vi "Get Spectrum.vi"(0 "waveform (V)":waveform(dbl), 1 "FFT window (7 Term B-Harris)":T1=8 items=["Rectangle"=0, "Hanning"=1, "Hamming"=2, "Blackman-Harris"=3, "Exact Blackman"=4, "Blackman"=5, "Flat Top"=6, "4 Term B-Harris "=7, "7 Term B-Harris"=8, "Low Sidelobe"=9, "Blackman Nuttall"=11, "Triangle"=30, "Bartlett-Hanning"=31, "Bohman"=32, "Parzen"=33, "Welch"=34, "Kaiser"=60, "Dolph-Chebyshev"=61, "Gaussian"=62], 11 "error in (no error)":errorcluster) -> (4 "power spectrum (dBm)":cluster{"f0":dbl, "df":dbl, "magnitude":dbl[]}, 15 "error out":errorcluster)   [LabVIEW 2021]
uses:
  <vilib>/Analysis/4window.llb/windowTd.ctl
  <vilib>/measure/maspectr.llb/FFT Power Spectrum and PSD for 1 Chan.vi
  <vilib>/measure/NI_MAPro.lvlib
  <vilib>/Analysis/NI_AALPro.lvlib
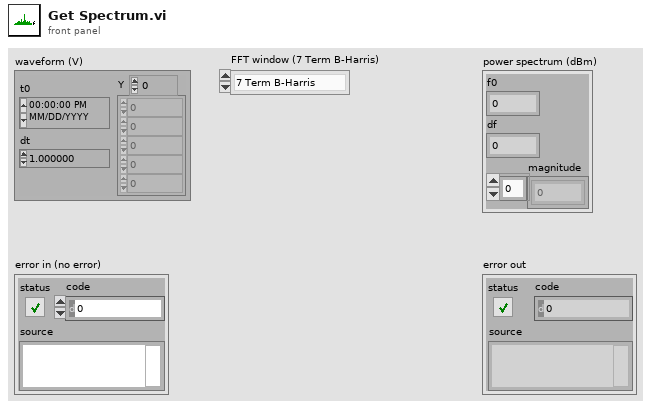
[diagram p1: front panel]
types:
  T1 = typedef "NI_AALPro.lvlib/windowTd.ctl" = u32
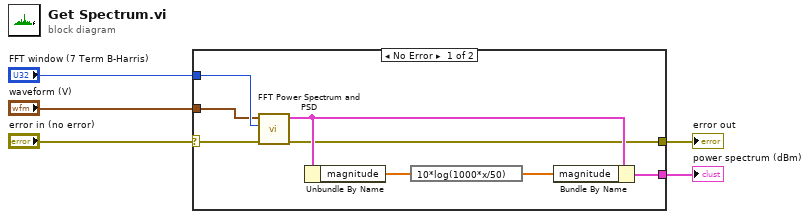
[diagram p0: block diagram]
diagram:
  n1 = case shown="No Error" "error in (no error)" {
    selector: "error in (no error)" -> [w9 w14]
    tunnel: [w12 _] -> w5
    tunnel: "waveform (V)" -> [w11 _]
    tunnel: [w7 w14] -> w2
    tunnel: "FFT window (7 Term B-Harris)" -> [w13 _]
    frame No Error {
      n2 = call-poly <vilib>:"FFT Power Spectrum and PSD.vi"("error in (no error)"=w9, "window"=w13, "time signal"=w11) -> ("error out"=w7:errorcluster, "Power Spectrum / PSD"=w8:cluster{"f0":dbl, "df":dbl, "magnitude":dbl[]})  [unwired: 5 in, 2 out]
      n3 = Unbundle By Name(w8) -> ("magnitude"=w10:dbl[])
      n4 = expression code="10*log(1000*x/50)"(w10) -> (w6:dbl[])
      n5 = Bundle By Name(cluster=w8, "magnitude"=w6) -> (w12:cluster{"f0":dbl, "df":dbl, "magnitude":dbl[]})
    }
    frame Error {
    }
  }
  "power spectrum (dBm)" <- w5
  "error out" <- w2
